vi "Database.GetProduct.vi"(8 "error in":errorcluster, 9 "serialNumberIn":u64, 10 "RefNumIn":u64) -> (0 "error out":errorcluster, 2 "Prod exist?":bool)   [LabVIEW 2016]
uses:
  Database.Global.vi
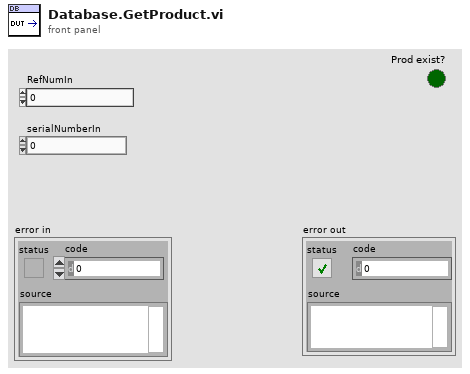
[diagram p1: front panel]
types:
  T1 = typedef "Database.Handler.Data.Sets.ctl" = cluster{"Enable":bool, "Export":bool, "ConnString":string, "Clients":i32}
  T2 = typedef "Database.Handler.Data.Status.ctl" = cluster{"Run":bool, "Handle":i32, "ConnTS":timestamp, "DbTime":timestamp, "DbTimeOffset":dbl}
  T3 = typedef "Database.Main.AccessLevel.ctl" = enum16{"connect only", "read only", "read/write"}
  T4 = typedef "ProdaNG.Identification.ctl" = cluster{"processId":i32, "systemId":i32, "processStepId":i32, "wabcoPartId":i32}
  T5 = typedef "ProdaNG.Product.ctl" = cluster{"c_id":string, "wabcoPartId":i32, "serialNumber":string, "comment":string, "individual":i32, "crProcessStepId":i32, "mdProcessStepId":i32, "crTime":string, "mdTime":string}
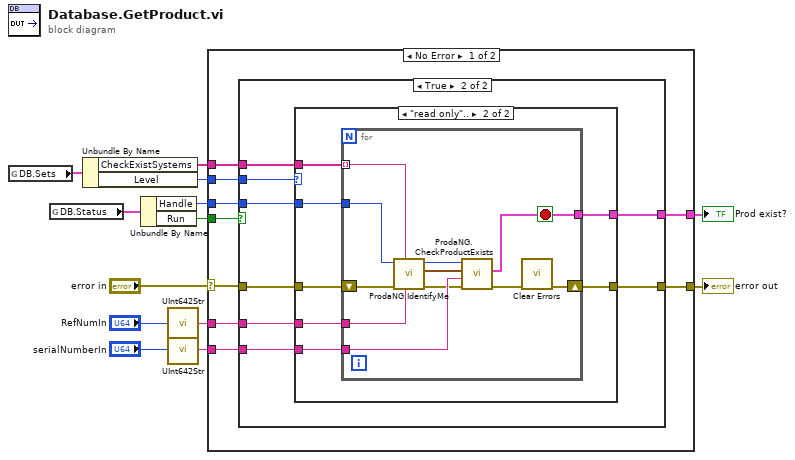
[diagram p0: block diagram]
diagram:
  n1 = global read "Database.Global.vi" "DB.Sets"() -> (w12:T1)
  n2 = global read "Database.Global.vi" "DB.Status"() -> (w13:T2)
  n3 = Unbundle By Name(w12) -> ("CheckExistSystems"=w11:string[], "Level"=w1:T3)
  n4 = Unbundle By Name(w13) -> ("Handle"=w10:i32, "Run"=w9:bool)
  n5 = call "UInt642Str.vi"("Numeric"="RefNumIn") -> ("string"=w5:string)
  n6 = call "UInt642Str.vi"("Numeric"="serialNumberIn") -> ("string"=w2:string)
  n7 = case shown="No Error" "error in" {
    selector: "error in" -> [w17 w51]
    tunnel: w11 -> [w22 _]
    tunnel: w10 -> [w21 _]
    tunnel: w9 -> [w20 _]
    tunnel: w5 -> [w19 _]
    tunnel: [w18 w51] -> w8
    tunnel: w2 -> [w16 _]
    tunnel: [w15 _] -> w6
    tunnel: w1 -> [w14 _]
    frame No Error {
      n8 = case shown="True" w20 {
        tunnel: w21 -> [_ w31]
        tunnel: w22 -> [_ w30]
        tunnel: w19 -> [_ w28]
        tunnel: w17 -> [w23 w29]
        tunnel: [w23 w26] -> w18
        tunnel: w16 -> [_ w27]
        tunnel: [_ w25] -> w15
        tunnel: w14 -> [_ w24]
        frame False {
        }
        frame True {
          # "First Process Step Parameter's description is sequence name!"
          n9 = case shown="\"read only\".." w24 {
            tunnel: w31 -> [_ w39]
            tunnel: w30 -> [_ w38]
            tunnel: w29 -> [w32 w37]
            tunnel: w28 -> [_ w36]
            tunnel: w27 -> [_ w35]
            tunnel: [w32 w34] -> w26
            tunnel: [_ w33] -> w25
            frame "connect only", Default {
            }
            frame "read only".. {
              n10 = for {
                tunnel: w39 -> [w50]
                tunnel: w38 -> [w49] mode=indexing
                tunnel: w36 -> [w47]
                tunnel: w35 -> [w46]
                tunnel: [w40] -> w33
                shift-right: [w44] -> w34
                shift-left: w37 -> [w48]
                stop <- w40 stop-if-true
                n11 = call "ProdaNG.IdentifyMe.vi"("wabcoNumber"=w47, "systemName"=w49, "error in"=w48, "dbHandleIn"=w50) -> ("error out"=w42:errorcluster, "Identification"=w41:T4, "dbHandle"=w43:i32)  [unwired: 5 in]
                n12 = call "ProdaNG.CheckProductExists.vi"("error in (no error)"=w42, "serialNumber"=w46, "ID"=w41, "dbHandle"=w43) -> ("error out"=w45:errorcluster, "ProductID"=w40:T5)  [unwired: 3 in, 3 out]
                n13 = call <vilib>:"Clear Errors.vi"("error in (no error)"=w45) -> ("error out"=w44:errorcluster)  [unwired: 5 in, 1 out]
              }
            }
          }
        }
      }
    }
    frame Error {
    }
  }
  "error out" <- w8
  "Prod exist?" <- w6
